vi "Write Force Sensor Settings.vi"(10 "Force Sensor Settings":T1={"ADC Channel"=1, "Reference Voltage Vref"=0.0} {"Reference Voltage Vref" min=-10.0 max=10.0 format="%.3f"}, 11 "Model in":refnum<class "Model.lvclass">) -> (3 "Model out":refnum<class "Model.lvclass">)   [LabVIEW 2015, in "Model.lvclass"]
uses:
  Model.lvclass
  Typedefs/ForceSensorSettings.ctl
  Model.lvclass/Model.ctl
  Typedefs/FAMTTypedefs.lvlib
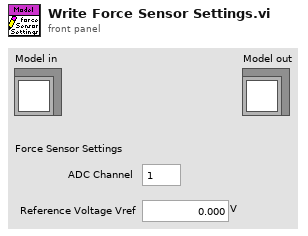
[diagram p1: front panel]
types:
  T1 = typedef "FAMTTypedefs.lvlib/ForceSensorSettings.ctl" = cluster{"ADC Channel":u8, "Reference Voltage Vref":dbl[unit]}
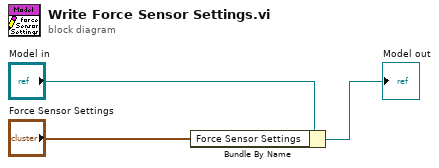
[diagram p0: block diagram]
diagram:
  n1 = Bundle By Name(cluster="Model in", "Force Sensor Settings"="Force Sensor Settings") -> (→"Model out":refnum<class "Model.lvclass">)
